vi "Map to VArray of Clusters__ogtk.vi"(8 "error in":errorcluster, 11 "Map":variant) -> (0 "error out":errorcluster, 3 "Array of Clusters (key-value)":variant)   [LabVIEW 2023, in "openg_variant.lvlib"]
uses:
  openg_variant.lvlib
panel:
  # "EXPERIMENTAL"
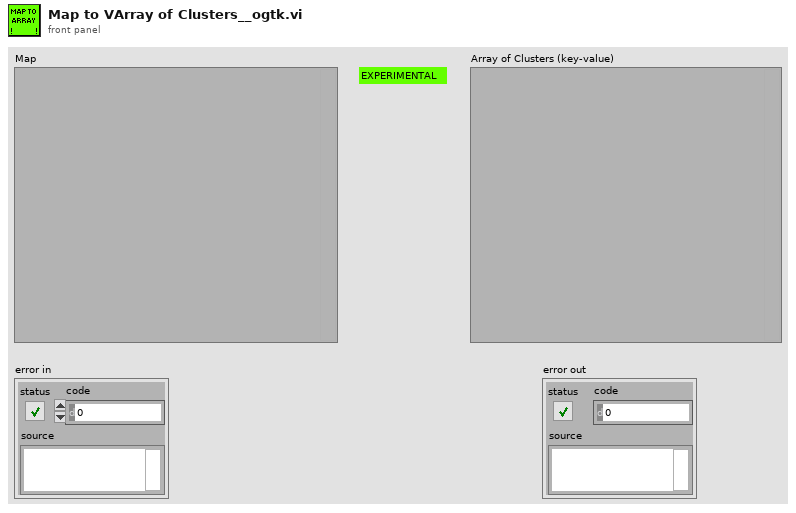
[diagram p1: front panel]
types:
  T1 = typedef "openg_variant.lvlib/Type Descriptor__ogtk.ctl" = i16[]
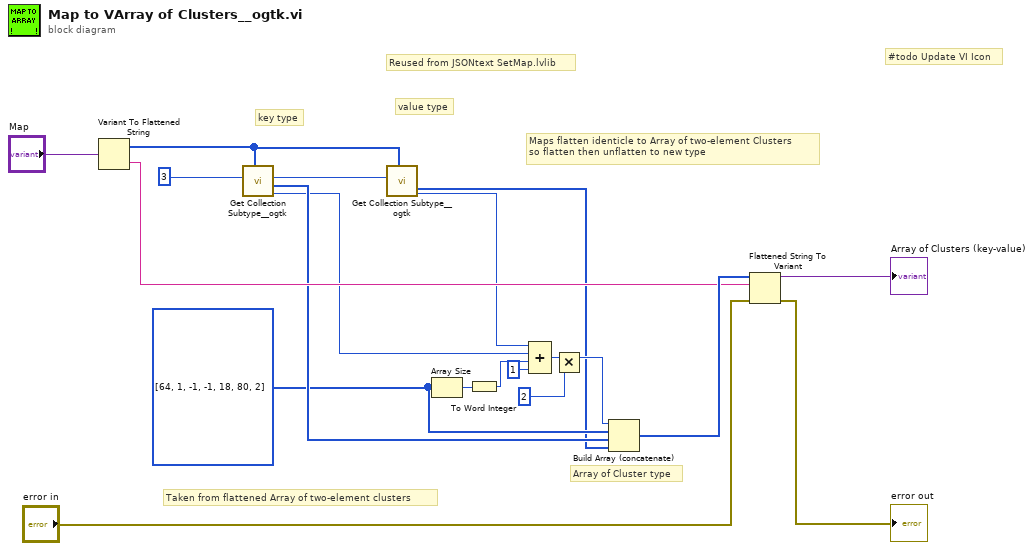
[diagram p0: block diagram]
diagram:
  w11 = i16[] [64, 1, -1, -1, 18, 80, 2] ("type string 7")
  # "#todo Update VI Icon"
  # "Reused from JSONtext SetMap.lvlib"
  # "Taken from flattened Array of two-element clusters"
  # "Maps flatten identicle to Array of two-element Clusters\nso flatten then unflatten to new type"
  # "value type"
  # "key type"
  # "Array of Cluster type"
  n1 = Variant To Flattened String(Variant="Map") -> (data string=w13:string, 1:w3:i16[])
  n2 = call "Get Collection Subtype__ogtk.vi"("Type Descriptor"=w3, "Offset In"=i16 3 ("index")) -> ("Size"=w5:i16, "subtype"=w12:T1, "Offset out"=w4:i16)  [unwired: 7 in]
  n3 = call "Get Collection Subtype__ogtk.vi"("Type Descriptor"=w3, "Offset In"=w4) -> ("Size"=w1:i16, "subtype"=w2:T1)  [unwired: 7 in, 1 out]
  n4 = Array Size(array=w11) -> (size(s)=w10:i32)
  n5 = To Word Integer(number=w10) -> (16bit integer=w8:i16)
  n6 = Compound Arithmetic op=ADD(w1, w5, w8, i16 1 ("value")) -> (w9:i16)
  n7 = Multiply(x=w9, y=i16 2) -> (x*y=w15:i16)
  n8 = Build Array (concatenate)(w15, w11, w12, w2) -> (w14:T1)
  n9 = Flattened String To Variant(4:"error in", 6:w13, 7:w14) -> (0:→"error out":errorcluster, 3:→"Array of Clusters (key-value)":variant)
